vi "W9EO82,FBO8PP_3.vi"() -> ()   [LabVIEW 2021]
panel:
  in  "Gomb":bool
  out "Boolean":bool
  out "sum":i64
  out "Array":i64[](array[numeric])
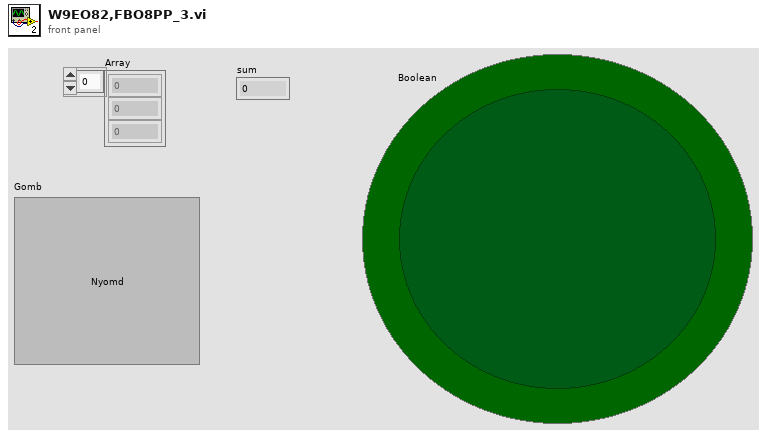
[diagram p1: front panel]
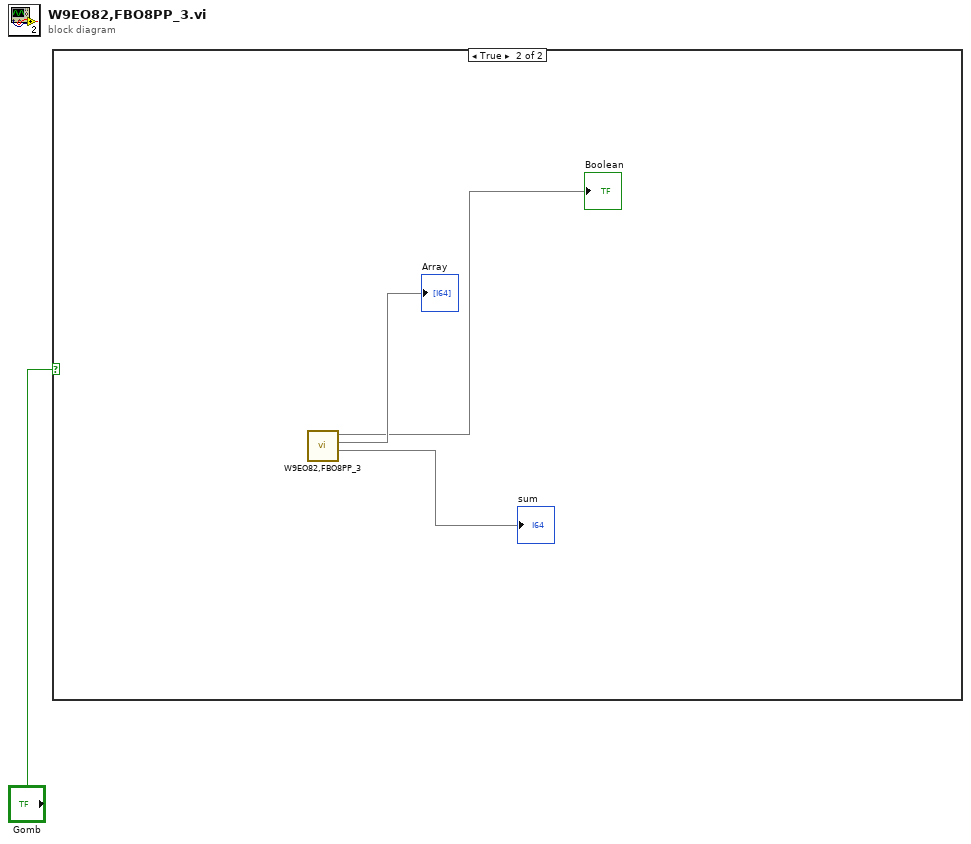
[diagram p0: block diagram]
diagram:
  n1 = case shown="True" "Gomb" {
    frame False {
    }
    frame True {
      n2 = call "W9EO82,FBO8PP_3.vi"() -> (1:→"sum", 2:→"Array", 3:→"Boolean")  [unwired: 9 in]
    }
  }
